vi "LidarParseTransformAndSend.vi"(1 "Raphael_Offsets":T1={"x_offset"=2000, "y_offset"=-450, "z_offset"=1000, "Theta_z"=-45.0, "Theta_y"=0.0} {"Theta_y" format="%.10g"; "Theta_z" format="%.10g"}, 2 "SelectLIDAR":enum16{"Raphael", "Leonardo"}(ring), 3 "Leonardo_Offsets":T1={"x_offset"=2000, "y_offset"=450, "z_offset"=1000, "Theta_z"=45.0, "Theta_y"=0.0} {"Theta_y" format="%.10g"; "Theta_z" format="%.10g"}) -> (0 "New Point?":bool)   [LabVIEW 2010]
doc: "LidarParseTransformAndSend.vi parses the byte string read in from the LIDAR, transforms it into robot coordinates, and pushes it to the PC.\n\n*Note - currently all offsets are set to default on the front panel.\n\n<b>Inputs</b>\nSelectLIDAR - select LIDAR from which to read data\n\nLeonardo_Offsets:\nx_offset - x offset of Leonardo in the robot's frame in mm\ny_offset - y offset of Leonardo in the robot's frame in mm\nz_offset - z offset of Leonardo in the robot's frame in mm\nTheta_y - pitch angle of Leonardo in degrees below horizontal\nTheta_z - yaw angle of Leonardo in degrees left of forward\n\nRaphael_Offsets:\nx_offset - x offset of Raphael in the robot's frame in mm\ny_offset - y offset of Raphael in the robot's frame in mm\nz_offset - z offset of Raphael in the robot's frame in mm\nTheta_y - pitch angle of Raphael in degrees below horizontal\nTheta_z - yaw angle of Raphael in degrees left of forward\n\n\n<b>Outputs</b>\nNew Point? - boolean to indicate if a new data point has been parsed"
uses:
  Type Defs/LidarOffsets.ctl
  <vilib>/rvi/DataTransferAndStorage/Container/XNode/niFpgaContainer.xnode
  <vilib>/rvi/DataTransferAndStorage/Container/Common/niFpgaTransferTypeControl.ctl
  <vilib>/rvi/FIFO/Fifo_Types/niFpgaFifoControlLogicControl.ctl
  <vilib>/rvi/DataTransferAndStorage/Container/Common/niFpgaContainerMethod.ctl
  <vilib>/rvi/DataTransferAndStorage/Container/Common/niFpgaContainerMetaDataKey.ctl
  <vilib>/rvi/DataTransferAndStorage/FIFO/niFpgaPeerToPeerStreamState.ctl
  <vilib>/rvi/DataTransferAndStorage/Container/Common/niFpgaContainerExecOnDevCompGetState.vi
  <vilib>/rvi/FIFO/Fifo_Resource/nirvififoEmulationSetSize.vi
  <vilib>/rvi/DataTransferAndStorage/Container/Common/niFpgaContainerGetUniqueNameForEmu.vi
  <vilib>/rvi/interface/RandomDataEmulation/nirviRandomDataFPGAFIFO.vi
  <vilib>/rvi/interface/RandomDataEmulation/niFpgaRandomDataHandleErrors.vi
  <vilib>/rvi/eio/common/nirviEmuReportErrorAndStop.vi
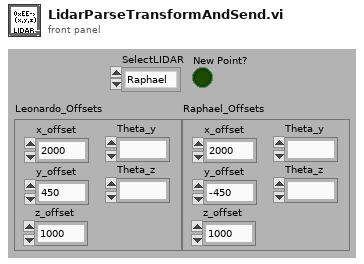
[diagram p1: front panel]
types:
  T1 = typedef "LidarOffsets.ctl" = cluster{"x_offset":i16, "y_offset":i16, "z_offset":i16, "Theta_z":fxp<+/-,16,9>, "Theta_y":fxp<+/-,16,9>}
  T2 = enum16{"confirm check sum", "check status byte", "read measured values", "confirm measurement", "confirm command", "read message length", "read address", "wait for \"02\""}
  T3 = typedef "niFpgaFifoControlLogicControl.ctl" = enum16{"Slice Fabric", "Target Optimal", "Built-in"}
  T4 = typedef "niFpgaContainerMethod.ctl" = enum16{"<none>", "write", "read", "clear", "getNumberOfElementsToWrite", "getNumberOfElementsToRead", "enable", "disable", "flushAndDisable", "getStreamState", "readA", "readB", "dramWrite", "dramWriteWithByteEnables", "dramRequestData", "dramRetrieveData"}
  T5 = typedef "niFpgaTransferTypeControl.ctl" = enum16{"Target-Scoped", "Host to Target - DMA", "Target to Host - DMA", "Peer to Peer Reader", "Peer to Peer Writer", "Bidirectional"}
  T6 = typedef "niFpgaPeerToPeerStreamState.ctl" = enum16{"Unlinked", "Disabled", "Enabled", "Flushing"}
  T7 = typedef "niFpgaContainerMetaDataKey.ctl" = enum16{"FPGA FIFO", "FPGA Memory", "FPGA Register"}
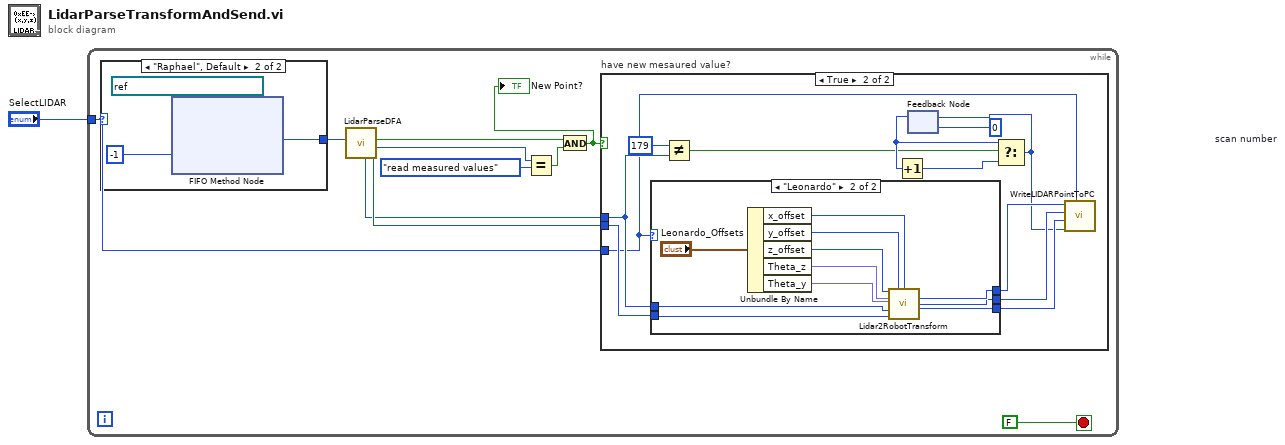
[diagram p0: block diagram]
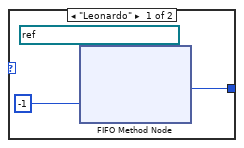
[diagram p2: hidden frame]
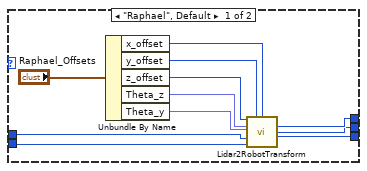
[diagram p4: hidden frame]
diagram:
  n1 = while {
    tunnel: "SelectLIDAR" -> [w4]
    stop <- FALSE stop-if-true
    n2 = case shown="\"Raphael\", Default" w4 {
      tunnel: [w14 w334] -> w2
      frame "Leonardo" {
        n3 = xnode ("FIFO Method Node")("Timeout"=-1, "FIFO In"=refnum<k21> "LIDARLeonardoReadFIFO" ("LIDAR Read FIFO 2")) -> ("Element"=w14:u8)  [unwired: 2 out]
      }
      frame "Raphael", Default {
        n4 = xnode ("FIFO Method Node")("Timeout"=-1, "FIFO In"=refnum<k21> "LIDARRaphaelReadFIFO" ("LIDAR Read FIFO 2")) -> ("Element"=w334:u8)  [unwired: 2 out]
      }
    }
    n5 = call "LidarParseDFA.vi"("LIDAR raw data"=w2) -> ("last measured value"=w11:u16, "parser state"=w10:T2, "new value?"=w9:bool, "angle"=w6:u8)  [unwired: 7 in]
    n6 = Equal?(x=w10, y=T2."read measured values" ("parser state")) -> (x = y?=w7:bool)
    n7 = And(x=w9, y=w7) -> (x .and. y?=w3:bool)
    "New Point?" <- w3
    n8 = case "have new mesaured value?" shown="True" w3 {
      tunnel: w11 -> [_ w657]
      tunnel: w6 -> [_ w658]
      tunnel: w4 -> [_ w652]
      frame False {
      }
      frame True {
        n9 = case shown="\"Leonardo\"" w652 {
          tunnel: w658 -> [w670 w681]
          tunnel: w657 -> [w671 w682]
          tunnel: [w674 w685] -> w656
          tunnel: [w673 w684] -> w655
          tunnel: [w672 w683] -> w654
          frame "Raphael", Default {
            n10 = Unbundle By Name("Raphael_Offsets") -> ("x_offset"=w668:i16, "y_offset"=w667:i16, "z_offset"=w666:i16, "Theta_z"=w665:fxp<+/-,16,9>, "Theta_y"=w664:fxp<+/-,16,9>)
            n11 = call "Lidar2RobotTransform.vi"("z_offset"=w666, "y_offset"=w667, "x_offset"=w668, "Theta_z (deg +/-250)"=w665, "Theta_y (deg +/-250)"=w664, "Angle (deg 0:1:180)"=w670, "Range (mm)"=w671) -> ("X"=w674:i16, "Y"=w673:i16, "Z"=w672:i16)  [unwired: 6 in]
          }
          frame "Leonardo" {
            n12 = Unbundle By Name("Leonardo_Offsets") -> ("x_offset"=w679:i16, "y_offset"=w678:i16, "z_offset"=w677:i16, "Theta_z"=w676:fxp<+/-,16,9>, "Theta_y"=w675:fxp<+/-,16,9>)
            n13 = call "Lidar2RobotTransform.vi"("z_offset"=w677, "y_offset"=w678, "x_offset"=w679, "Theta_z (deg +/-250)"=w676, "Theta_y (deg +/-250)"=w675, "Angle (deg 0:1:180)"=w681, "Range (mm)"=w682) -> ("X"=w685:i16, "Y"=w684:i16, "Z"=w683:i16)  [unwired: 6 in]
          }
        }
        n14 = Not Equal?(x=u8 179, y=w658) -> (x != y?=w661:bool)
        n15 = feedback #1 "scan number"(u8 0 ("y")) -> (w663:u8)
        n16 = Increment(x=w663) -> (x+1=w662:u8)
        n17 = Select(t=w663, s=w661, f=w662) -> (s? t:f=w653:u8)
        n18 = feedback-in #1(w653) -> ()
        n19 = call "WriteLIDARPointToPC.vi"("SelectLIDAR"=w652, "count"=w653, "z"=w654, "y"=w655, "x"=w656) -> ()  [unwired: 6 in, 1 out]
      }
    }
  }
